vi "PM103 SCPI Example.vi"() -> ()   [LabVIEW 2013]
uses:
  <vilib>/regexp/Match Regular Expression.xnode
  <vilib>/ErrorRing/Error Ring.xnode
  <vilib>/Utility/error.llb/Error Cluster From Error Code.vi
panel:
  in  "stop":bool
  out "ARR LEN":i32
  out "rate":dbl format="%#.2f"
  out "count":i32
  out "time":u32
  out "error out":errorcluster
  in  "Tab Control":T1(tab)
  out "Chart":dbl(graph)
  in  "Scope Mode Array Length":i32=100
  out "Scope Mode Array [timestamp(us), power(W)]":cluster{u32, sgl}[](array[cluster])
  in  "Burst Mode Array Length":i32=100
  out "Burst Mode Array [timestamp(us), power(W)]":cluster{u32, sgl}[](array[cluster])
  out "Product Info":string
  # "Average Sampling Rate (Samples/s)"
  # "(range is 1 to 100)"
  # "I/O ports are 5 V TTL tolerant. The start of measurement is triggered on the rising edge of the TTL signal. In this example, the DIO1 is configured as IALT."
  # "(range is 1 to 100)"
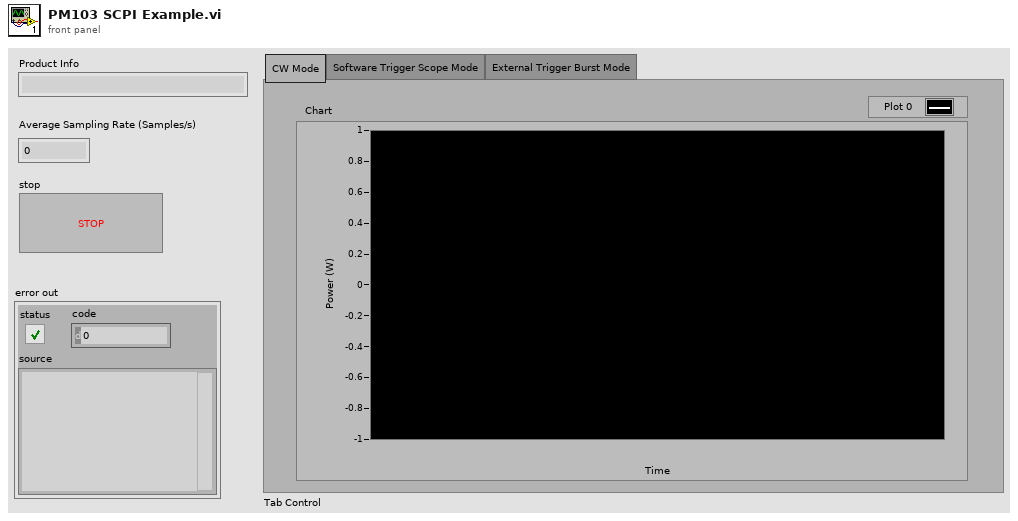
[diagram p1: front panel]
types:
  T1 = enum32{"CW Mode", "Software Trigger Scope Mode", "External Trigger Burst Mode"}
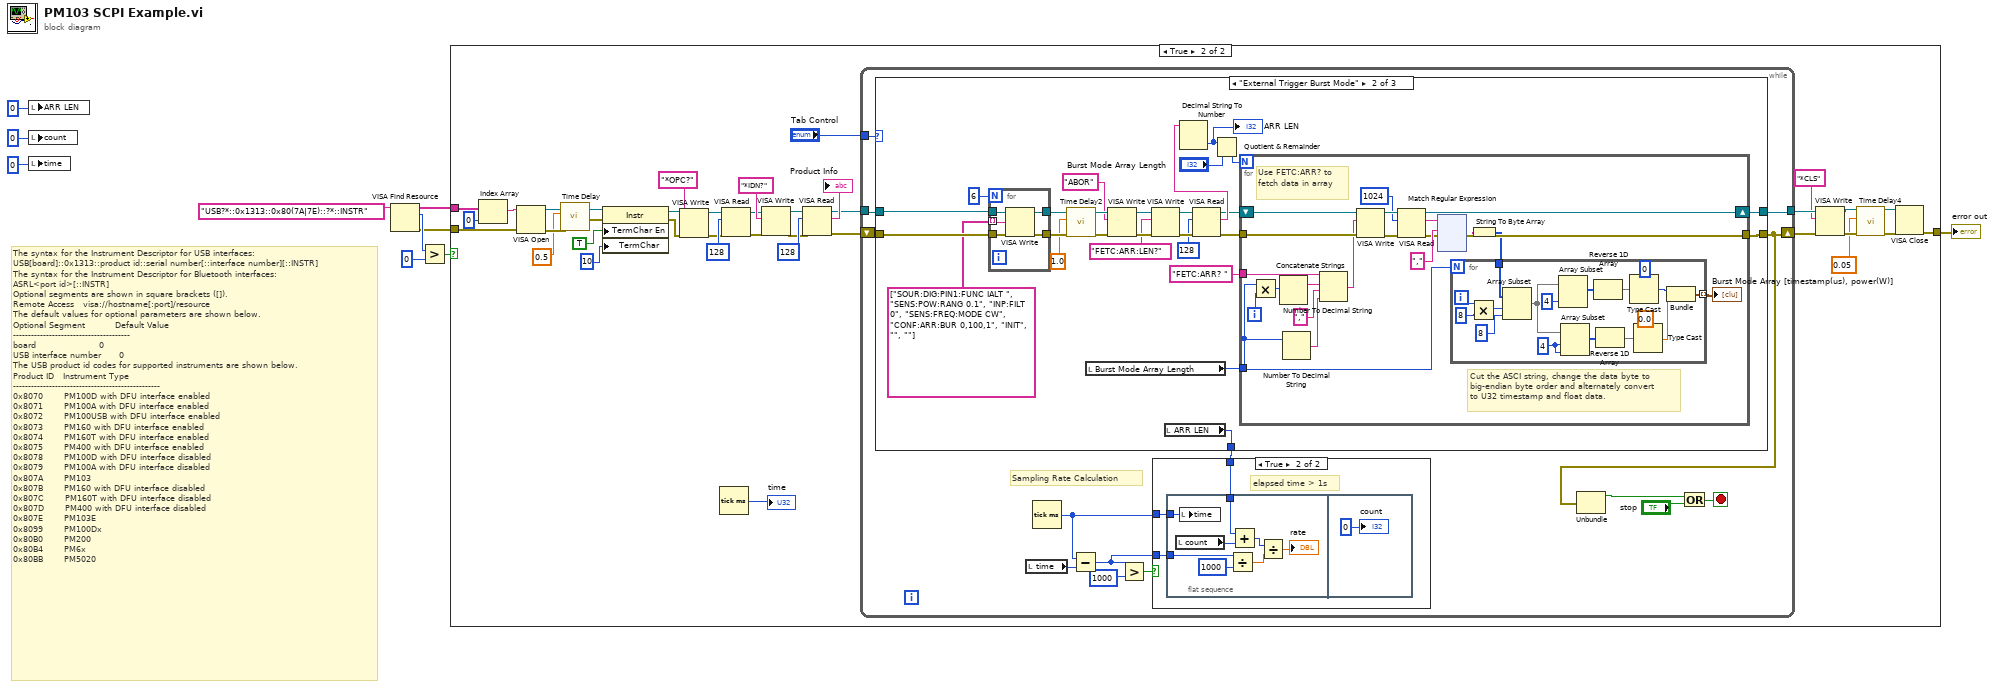
[diagram p0: block diagram]
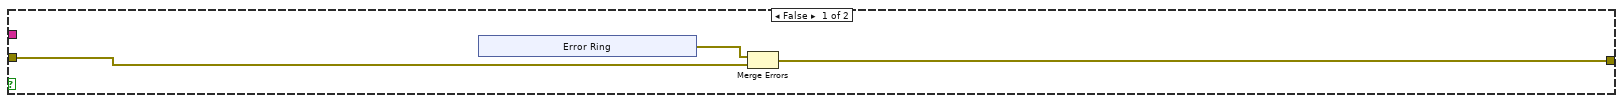
[diagram p2: hidden frame]
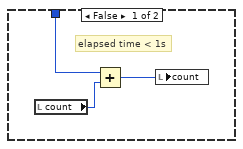
[diagram p3: hidden frame]
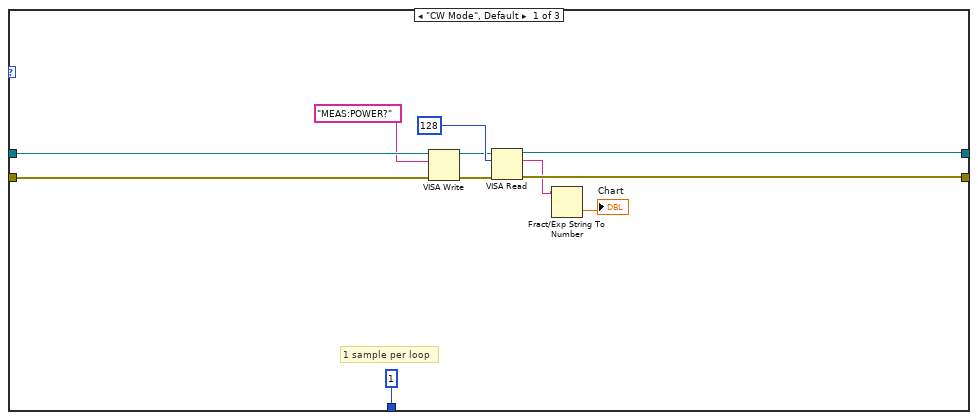
[diagram p4: hidden frame]
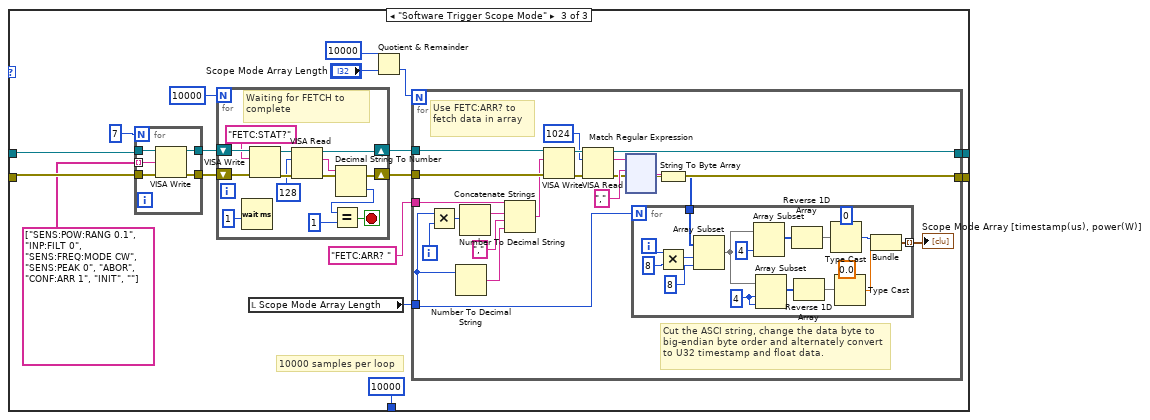
[diagram p5: hidden frame]
diagram:
  # "The syntax for the Instrument Descriptor for USB interfaces:\nUSB[board]::0x1313::product id::serial number[::interface number][::INSTR]\nThe syntax for the Instrument Descriptor for Bluetooth interfaces:\nASRL<port id>[::INSTR]\nOptional segments are shown in square brackets ([]).\nRemote Access   visa://hostname[:port]/resource\nThe default values for optional parameters are shown below.\nOptional Segment          Default Value\n---------------------------------------\nboard                     0\nUSB interface number      0\nThe USB product id codes for supported instruments are shown below.\nProduct ID   Instrument Type\n-------------------------------------------------\n0x8070       PM100D with DFU interface enabled\n0x8071       PM100A with DFU interface enabled\n0x8072       PM100USB with DFU interface enabled\n0x8073       PM160 with DFU interface enabled\n0x8074       PM160T with DFU interface enabled\n0x8075       PM400 with DFU interface enabled\n0x8078       PM100D with DFU interface disabled\n0x8079       PM100A with DFU interface disabled\n0x807A       PM103\n0x807B       PM160 with DFU interface disabled\n0x807C       PM160T with DFU interface disabled\n0x807D       PM400 with DFU interface disabled\n0x807E       PM103E\n0x8099       PM100Dx\n0x80B0       PM200\n0x80B4       PM6x\n0x80BB       PM5020"
  n1 = local write "ARR LEN"(0 ("ARR LEN")) -> ()
  n2 = local write "count"(0 ("loopCount")) -> ()
  n3 = local write "time"(u32 0 ("time")) -> ()
  n4 = VISA Find Resource(11:"USB?*::0x1313::0x80(7A|7E)::?*::INSTR" ("expression (\"?*\")")) -> (0:w4:errorcluster, 2:w9:u32, 3:w6:string[])  [unwired: 2 in]
  n5 = Greater?(x=w9, y=u32 0) -> (0:w7:bool)
  n6 = case shown="True" w7 {
    tunnel: w6 -> [_ w53]
    tunnel: [w13 w26] -> w5
    tunnel: w4 -> [w12 w38]
    frame False {
      n7 = xnode "Error Ring"() -> ("error out"=w11:errorcluster)
      n8 = Merge Errors(w11, w12) -> (w13:errorcluster)
    }
    frame True {
      n9 = Index Array(array=w53, index=0) -> (element=w39:string)
      n10 = VISA Open(error in (no error)=w38, VISA resource name=w39) -> (VISA resource name=w45:refnum<visa-resource-name>, error out=w48:errorcluster)  [unwired: 3 in]
      n11 = call "Time Delay"("error in (no error)"=w48, "Delay Time (s)"=0.5) -> ("error out"=w46:errorcluster)  [unwired: 9 in]
      n12 = property class="Instr"(reference=w45, error in=w46, "TermChar En"=TRUE ("Message Based Settings:Termination Character Enable"), "TermChar"=u8 10 ("Message Based Settings:Termination Character")) -> (reference out=w22:refnum<visa-resource-name>, error out=w21:errorcluster)
      n13 = VISA Write(VISA resource name=w22, write buffer="*OPC?", error in (no error)=w21) -> (VISA resource name out=w34:refnum<visa-resource-name>, error out=w19:errorcluster)  [unwired: 1 out]
      n14 = Tick Count (ms)() -> (millisecond timer value=→"time":u32)
      n15 = VISA Read(VISA resource name=w34, byte count=u32 128, error in (no error)=w19) -> (VISA resource name out=w33:refnum<visa-resource-name>, error out=w36:errorcluster)  [unwired: 2 out]
      n16 = VISA Write(VISA resource name=w33, write buffer="*IDN?", error in (no error)=w36) -> (VISA resource name out=w50:refnum<visa-resource-name>, error out=w25:errorcluster)  [unwired: 1 out]
      n17 = VISA Read(VISA resource name=w50, byte count=u32 128, error in (no error)=w25) -> (VISA resource name out=w42:refnum<visa-resource-name>, read buffer=→"Product Info":string, error out=w41:errorcluster)  [unwired: 1 out]
      n18 = while {
        tunnel: [w67] -> w31
        tunnel: w42 -> [w66]
        tunnel: "Tab Control" -> [w64]
        shift-right: [w56] -> w32
        shift-left: w41 -> [w65]
        stop <- w54 stop-if-true
        # "Sampling Rate Calculation"
        n19 = case shown="\"External Trigger Burst Mode\"" w64 {
          tunnel: [w90 w117 w293] -> w67
          tunnel: w66 -> [w92 w118 w294]
          tunnel: [w89 w119 w295] -> w56
          tunnel: w65 -> [w91 w116 w292]
          tunnel: [1 w115 10000 ("x")] -> w61
          frame "CW Mode", Default {
            # "1 sample per loop"
            n20 = VISA Write(VISA resource name=w92, write buffer="MEAS:POWER?", error in (no error)=w91) -> (VISA resource name out=w84:refnum<visa-resource-name>, error out=w83:errorcluster)  [unwired: 1 out]
            n21 = VISA Read(VISA resource name=w84, byte count=u32 128, error in (no error)=w83) -> (VISA resource name out=w90:refnum<visa-resource-name>, read buffer=w87:string, error out=w89:errorcluster)  [unwired: 1 out]
            n22 = Fract/Exp String To Number(string=w87) -> (number=→"Chart":dbl)  [unwired: 3 in, 1 out]
          }
          frame "External Trigger Burst Mode" {
            n23 = for {
              N: 6 -> [_]
              tunnel: string[] ["SOUR:DIG:PIN1:FUNC IALT ", "SENS:POW:RANG 0.1", "INP:FILT 0", "SENS:FREQ:MODE CW", "CONF:ARR:BUR 0,100,1", "INIT", "", ""] -> [w276] mode=indexing
              tunnel: w116 -> [w278]
              tunnel: w118 -> [w277]
              tunnel: [w275] -> w112
              tunnel: [w274] -> w109
              n24 = VISA Write(VISA resource name=w277, write buffer=w276, error in (no error)=w278) -> (VISA resource name out=w274:refnum<visa-resource-name>, error out=w275:errorcluster)  [unwired: 1 out]
            }
            n25 = call "Time Delay2"("error in (no error)"=w112, "Delay Time (s)"=1.0) -> ("error out"=w110:errorcluster)  [unwired: 9 in]
            n26 = local read "Burst Mode Array Length"() -> (w94:i32)
            n27 = VISA Write(VISA resource name=w109, write buffer="ABOR", error in (no error)=w110) -> (VISA resource name out=w106:refnum<visa-resource-name>, error out=w107:errorcluster)  [unwired: 1 out]
            n28 = VISA Write(VISA resource name=w106, write buffer="FETC:ARR:LEN?", error in (no error)=w107) -> (VISA resource name out=w103:refnum<visa-resource-name>, error out=w104:errorcluster)  [unwired: 1 out]
            n29 = local read "ARR LEN"() -> (w115:i32)
            n30 = VISA Read(VISA resource name=w103, byte count=u32 128, error in (no error)=w104) -> (VISA resource name out=w99:refnum<visa-resource-name>, read buffer=w101:string, error out=w100:errorcluster)  [unwired: 1 out]
            n31 = Decimal String To Number(string=w101) -> (number=w97:i32)  [unwired: 2 in, 1 out]
            "ARR LEN" <- w97
            n32 = Quotient & Remainder(x=w97, y="Burst Mode Array Length") -> (floor(x/y)=w95:i32)  [unwired: 1 out]
            n33 = for {
              N: w95 -> [_]
              tunnel: w100 -> [w139]
              tunnel: "FETC:ARR? " ("write buffer") -> [w130]
              tunnel: [w124] -> w119
              tunnel: w94 -> [w121]
              shift-right: [w125] -> w117
              shift-left: w99 -> [w137]
              i -> [w128]
              # "Cut the ASCI string, change the data byte to big-endian byte order and alternately convert to U32 timestamp and float data."
              # "Use FETC:ARR? to fetch data in array"
              n34 = Multiply(x=w121, y=w128) -> (x*y=w132:i32)
              n35 = Number To Decimal String(number=w132) -> (decimal integer string=w134:string)  [unwired: 1 in]
              n36 = Number To Decimal String(number=w121) -> (decimal integer string=w131:string)  [unwired: 1 in]
              n37 = Concatenate Strings(w130, w134, "," ("string"), w131) -> (w129:string)
              n38 = VISA Write(VISA resource name=w137, write buffer=w129, error in (no error)=w139) -> (VISA resource name out=w136:refnum<visa-resource-name>, error out=w138:errorcluster)  [unwired: 1 out]
              n39 = VISA Read(VISA resource name=w136, byte count=u32 1024, error in (no error)=w138) -> (VISA resource name out=w125:refnum<visa-resource-name>, read buffer=w127:string, error out=w124:errorcluster)  [unwired: 1 out]
              n40 = xnode "Match Regular Expression"("input string"=w127, "regular expression"=",") -> ("after match"=w123:string)  [unwired: 4 in, 4 out]
              n41 = String To Byte Array(string=w123) -> (unsigned byte array=w122:u8[])
              n42 = for {
                N: w121 -> [_]
                tunnel: w122 -> [w156]
                tunnel: [w144] -> w120 mode=indexing
                i -> [w154]
                w149 = 4 ("index")
                n43 = Multiply(x=w154, y=8) -> (x*y=w155:i32)
                n44 = Array Subset(array=w156, index=w155, length=8) -> (w150:u8[])
                n45 = Array Subset(array=w150, length=4) -> (w143:u8[])  [unwired: 1 in]
                n46 = Array Subset(array=w150, index=w149, length=w149) -> (w141:u8[])
                n47 = Reverse 1D Array(array=w143) -> (reversed array=w142:u8[])
                n48 = Reverse 1D Array(array=w141) -> (reversed array=w140:u8[])
                n49 = Type Cast(type=u32 0, x=w142) -> (*(type *) &x=w146:u32)
                n50 = Type Cast(type=sgl 0.0, x=w140) -> (*(type *) &x=w145:sgl)
                n51 = Bundle(w146, w145) -> (w144:cluster{u32, sgl})  [unwired: 1 in]
              }
              "Burst Mode Array [timestamp(us), power(W)]" <- w120
            }
          }
          frame "Software Trigger Scope Mode" {
            # "10000 samples per loop"
            n52 = for {
              N: 7 -> [_]
              tunnel: w292 -> [w467]
              tunnel: w294 -> [w466]
              tunnel: [w465] -> w285
              tunnel: [w464] -> w289
              tunnel: string[] ["SENS:POW:RANG 0.1", "INP:FILT 0", "SENS:FREQ:MODE CW", "SENS:PEAK 0", "ABOR", "CONF:ARR 1", "INIT", ""] -> [w463] mode=indexing
              n53 = VISA Write(VISA resource name=w466, write buffer=w463, error in (no error)=w467) -> (VISA resource name out=w464:refnum<visa-resource-name>, error out=w465:errorcluster)  [unwired: 1 out]
            }
            n54 = for {
              N: 10000 -> [_]
              shift-right: [w303] -> w287
              shift-left: w289 -> [w308]
              shift-right: [w302] -> w286
              shift-left: w285 -> [w306]
              stop <- w297 stop-if-true
              # "Waiting for FETCH to complete"
              n55 = Wait (ms)(milliseconds to wait=u32 1) -> ()  [unwired: 1 out]
              n56 = VISA Write(VISA resource name=w308, write buffer="FETC:STAT?", error in (no error)=w306) -> (VISA resource name out=w304:refnum<visa-resource-name>, error out=w305:errorcluster)  [unwired: 1 out]
              n57 = VISA Read(VISA resource name=w304, byte count=u32 128, error in (no error)=w305) -> (VISA resource name out=w303:refnum<visa-resource-name>, read buffer=w300:string, error out=w302:errorcluster)  [unwired: 1 out]
              n58 = Decimal String To Number(string=w300) -> (number=w299:i32)  [unwired: 2 in, 1 out]
              n59 = Equal?(x=w299, y=1) -> (x = y?=w297:bool)
            }
            n60 = local read "Scope Mode Array Length"() -> (w280:i32)
            n61 = Quotient & Remainder(x=10000, y="Scope Mode Array Length") -> (floor(x/y)=w283:i32)  [unwired: 1 out]
            n62 = for {
              N: w283 -> [_]
              tunnel: w286 -> [w328]
              tunnel: w287 -> [w326]
              tunnel: "FETC:ARR? " ("write buffer") -> [w324]
              tunnel: [w320] -> w293
              tunnel: w280 -> [w309]
              tunnel: [w313] -> w295
              i -> [w317]
              # "Cut the ASCI string, change the data byte to big-endian byte order and alternately convert to U32 timestamp and float data."
              # "Use FETC:ARR? to fetch data in array"
              n63 = Multiply(x=w309, y=w317) -> (x*y=w318:i32)
              n64 = Number To Decimal String(number=w309) -> (decimal integer string=w316:string)  [unwired: 1 in]
              n65 = Number To Decimal String(number=w318) -> (decimal integer string=w323:string)  [unwired: 1 in]
              n66 = Concatenate Strings(w324, w323, "," ("string"), w316) -> (w322:string)
              n67 = VISA Write(VISA resource name=w326, write buffer=w322, error in (no error)=w328) -> (VISA resource name out=w325:refnum<visa-resource-name>, error out=w327:errorcluster)  [unwired: 1 out]
              n68 = VISA Read(VISA resource name=w325, byte count=u32 1024, error in (no error)=w327) -> (VISA resource name out=w320:refnum<visa-resource-name>, read buffer=w312:string, error out=w313:errorcluster)  [unwired: 1 out]
              n69 = xnode "Match Regular Expression"("input string"=w312, "regular expression"=",") -> ("after match"=w314:string)  [unwired: 4 in, 4 out]
              n70 = String To Byte Array(string=w314) -> (unsigned byte array=w311:u8[])
              n71 = for {
                N: w309 -> [_]
                tunnel: w311 -> [w345]
                tunnel: [w333] -> w310 mode=indexing
                i -> [w343]
                w338 = 4 ("index")
                n72 = Multiply(x=w343, y=8) -> (x*y=w344:i32)
                n73 = Array Subset(array=w345, index=w344, length=8) -> (w339:u8[])
                n74 = Array Subset(array=w339, length=4) -> (w332:u8[])  [unwired: 1 in]
                n75 = Array Subset(array=w339, index=w338, length=w338) -> (w330:u8[])
                n76 = Reverse 1D Array(array=w332) -> (reversed array=w331:u8[])
                n77 = Reverse 1D Array(array=w330) -> (reversed array=w329:u8[])
                n78 = Type Cast(type=u32 0, x=w331) -> (*(type *) &x=w335:u32)
                n79 = Type Cast(type=sgl 0.0, x=w329) -> (*(type *) &x=w334:sgl)
                n80 = Bundle(w335, w334) -> (w333:cluster{u32, sgl})  [unwired: 1 in]
              }
              "Scope Mode Array [timestamp(us), power(W)]" <- w310
            }
          }
        }
        n81 = local read "time"() -> (w60:u32)
        n82 = Tick Count (ms)() -> (millisecond timer value=w62:u32)
        n83 = Subtract(x=w62, y=w60) -> (x-y=w59:u32)
        n84 = Greater?(x=w59, y=u32 1000) -> (0:w55:bool)
        n85 = case shown="True" w55 {
          tunnel: w62 -> [_ w73]
          tunnel: w61 -> [w69 w71]
          tunnel: w59 -> [_ w72]
          frame False {
            # "elapsed time < 1s"
            n86 = local read "count"() -> (w70:i32)
            n87 = Add(x=w69, y=w70) -> (x+y=w68:i32)
            n88 = local write "count"(w68) -> ()
          }
          frame True {
            # "elapsed time > 1s"
            n89 = flat-sequence {
              tunnel: w73 -> [w81]
              tunnel: w72 -> [w78]
              tunnel: w71 -> [w74]
              frame #0 {
                n90 = local read "count"() -> (w75:i32)
                n91 = local write "time"(w81) -> ()
                n92 = Divide(x=w78, y=u32 1000) -> (x/y=w79:dbl)
                n93 = Add(x=w74, y=w75) -> (x+y=w76:i32)
                n94 = Divide(x=w76, y=w79) -> (x/y=→"rate":dbl)
              }
              frame #1 {
                "count" <- 0 ("count")
              }
            }
          }
        }
        n95 = Unbundle(w56) -> ("status"=w57:bool)  [unwired: 2 out]
        n96 = Or(x=w57, y="stop") -> (x .or. y?=w54:bool)
      }
      n97 = VISA Write(VISA resource name=w31, write buffer="*CLS", error in (no error)=w32) -> (VISA resource name out=w30:refnum<visa-resource-name>, error out=w28:errorcluster)  [unwired: 1 out]
      n98 = call "Time Delay4"("error in (no error)"=w28, "Delay Time (s)"=0.05) -> ("error out"=w27:errorcluster)  [unwired: 9 in]
      n99 = VISA Close(VISA resource name=w30, error in (no error)=w27) -> (error out=w26:errorcluster)
    }
  }
  "error out" <- w5
